vi "Read.vi"(8 "error in (no error)":errorcluster, 11 "Agilent DSO-X 3032A in":refnum<class "Agilent DSO-X 3032A.lvclass">) -> (0 "error out":errorcluster, 1 "timed out?":bool, 2 "Data":refnum<class "AbstractData.lvclass">, 3 "Agilent DSO-X 3032A out":refnum<class "Agilent DSO-X 3032A.lvclass">)   [LabVIEW 2014, in "Agilent DSO-X 3032A.lvclass"]
uses:
  Agilent DSO-X 3032A.lvclass
  Framework/Model/Data/AbstractData/AbstractData.lvclass
  Agilent DSO-X 3032A.lvclass/Agilent DSO-X 3032A.ctl
  Framework/Model/Data/Data1D/Data1D.lvclass
  Framework/Interfaces/Observable Actor/Observable Actor.lvclass
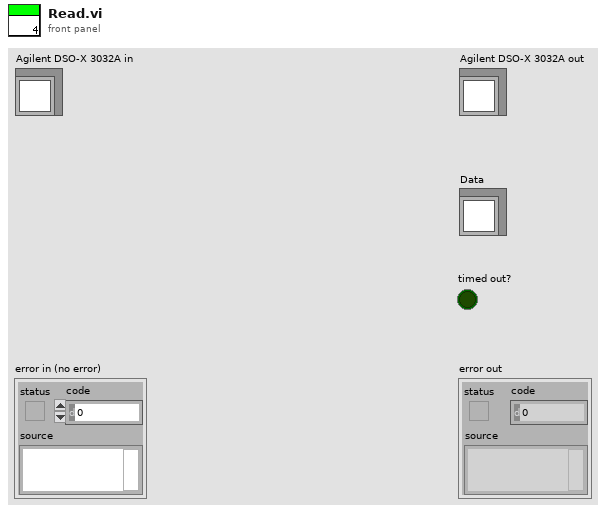
[diagram p1: front panel]
types:
  T1 = typedef "Agilent DSO-X 3032A.lvclass/Channel Settings.ctl" = cluster{"Dt":dbl, "#samples":i32, "t0":dbl}
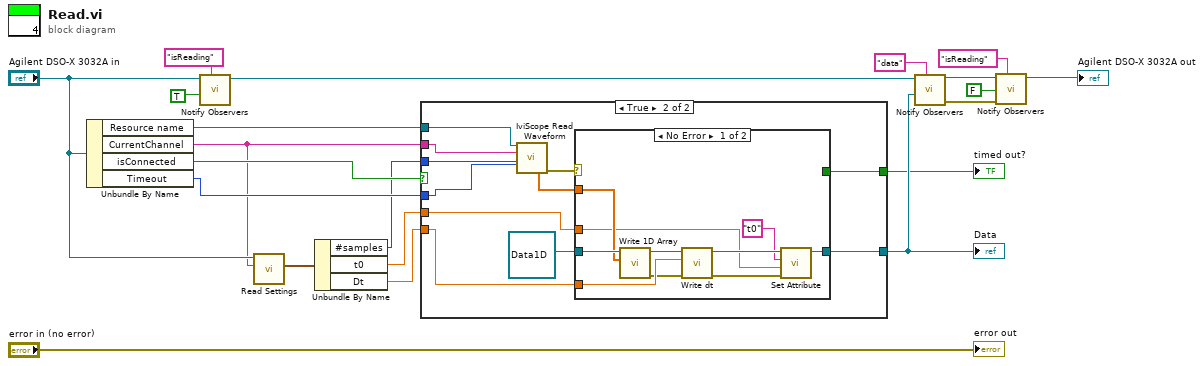
[diagram p0: block diagram]
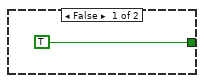
[diagram p2: hidden frame]
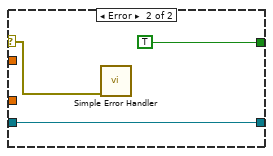
[diagram p3: hidden frame]
diagram:
  n1 = Unbundle By Name("Agilent DSO-X 3032A in") -> ("Resource name"=w21:refnum<k15>, "CurrentChannel"=w1:string, "isConnected"=w20:bool, "Timeout"=w19:i32)
  n2 = call "Notify Observers.vi"("name"="isReading", "value"=TRUE, "Observable Actor in"="Agilent DSO-X 3032A in") -> ("Observable Actor out"=w7:refnum<class "Agilent DSO-X 3032A.lvclass">)  [unwired: 7 in, 1 out]
  n3 = call "Read Settings.vi"("Channel"=w1, "Agilent DSO-X 3032A in"="Agilent DSO-X 3032A in") -> ("Settings"=w5:T1)  [unwired: 7 in, 2 out]
  n4 = Unbundle By Name(w5) -> ("#samples"=w2:i32, "t0"=w3:dbl, "Dt"=w4:dbl)
  n5 = case shown="True" w20 {
    tunnel: [_ w27] -> w18
    tunnel: w2 -> [_ w31]
    tunnel: w21 -> [_ w33]
    tunnel: w19 -> [_ w23]
    tunnel: w1 -> [_ w32]
    tunnel: [TRUE w26] -> w16
    tunnel: w3 -> [_ w24]
    tunnel: w4 -> [_ w25]
    frame False {
    }
    frame True {
      n6 = call <vilib>:"IviScope Read Waveform.vi"("instrument handle"=w33, "channel name (\"CHANNEL1\")"=w32, "waveform size (0)"=w31, "maximum time (5000ms)"=w23) -> ("waveform array"=w29:dbl[], "error out"=w30:errorcluster)  [unwired: 6 in, 4 out]
      n7 = case shown="No Error" w30 {
        selector: w30 -> [_ w44]
        tunnel: w29 -> [w41 _]
        tunnel: refnum<class "Data1D.lvclass"> refnum ("Data1D.lvclass") -> [w43 w46]
        tunnel: [w37 w46] -> w27
        tunnel: w25 -> [w40 _]
        tunnel: [_ TRUE] -> w26
        tunnel: w24 -> [w34 _]
        frame No Error {
          n8 = call "Write 1D Array.vi"("1D Array"=w41, "Data1D in"=w43) -> ("error out"=w39:errorcluster, "Data1D out"=w42:refnum<class "Data1D.lvclass">)  [unwired: 8 in]
          n9 = call "Write dt.vi"("error in (no error)"=w39, "dt"=w40, "Data1D in"=w42) -> ("error out"=w35:errorcluster, "Data1D out"=w38:refnum<class "Data1D.lvclass">)  [unwired: 7 in]
          n10 = call-dynamic "Set Attribute.vi"("error in (no error)"=w35, "Value"=w34, "Name"="t0", "AbstractData in"=w38) -> ("AbstractData out"=w37:refnum<class "Data1D.lvclass">)  [unwired: 5 in, 2 out]
        }
        frame Error {
          n11 = call <vilib>:"Simple Error Handler.vi"("error in (no error)"=w44) -> ()  [unwired: 4 in, 5 out]
        }
      }
    }
  }
  "Data" <- w18
  "timed out?" <- w16
  n12 = call "Notify Observers.vi"("name"="data", "value"=w18, "Observable Actor in"=w7) -> ("error out"=w12:errorcluster, "Observable Actor out"=w13:refnum<class "Agilent DSO-X 3032A.lvclass">)  [unwired: 7 in]
  n13 = call "Notify Observers.vi"("name"="isReading", "error in (no error)"=w12, "value"=FALSE, "Observable Actor in"=w13) -> ("Observable Actor out"=→"Agilent DSO-X 3032A out":refnum<class "Agilent DSO-X 3032A.lvclass">)  [unwired: 6 in, 1 out]
  "error out" <- "error in (no error)"
